vi "calculator.vi"() -> ()   [LabVIEW 2017]
panel:
  in  "QIUET":bool
  in  "*":bool
  in  "MC":bool
  in  "MR":bool
  in  "M+":bool
  in  "MS":bool
  in  "1/X":bool
  in  "+/-":bool
  in  "sqt":bool
  in  ".":bool
  out "INPUT/OUTPUT":string
  in  "b":bool
  in  "c":bool
  in  "/":bool
  in  "-":bool
  in  "+":bool
  in  "0":bool
  in  "9":bool
  in  "6":bool
  in  "8":bool
  in  "5":bool
  in  "7":bool
  in  "4":bool
  in  "3":bool
  in  "2":bool
  in  "1":bool
  in  "=":bool
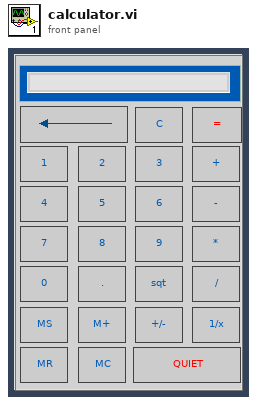
[diagram p1: front panel]
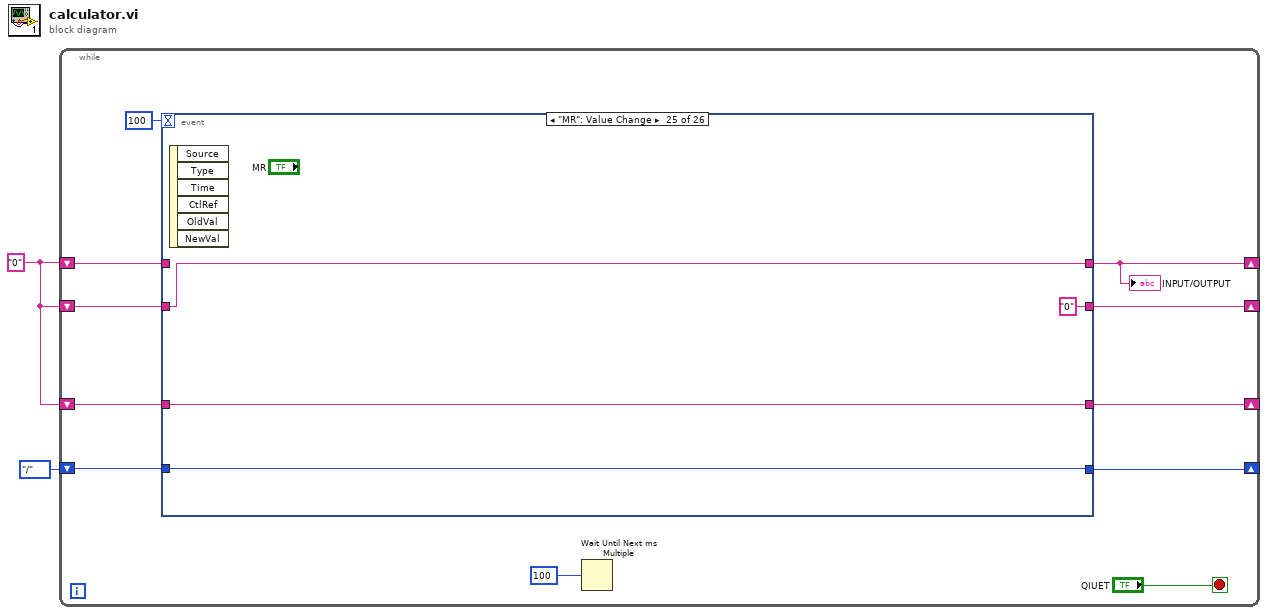
[diagram p0: block diagram]
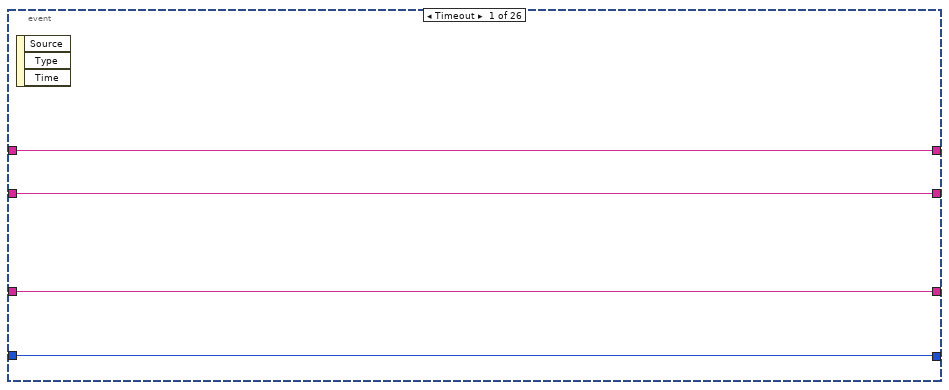
[diagram p2: hidden frame]
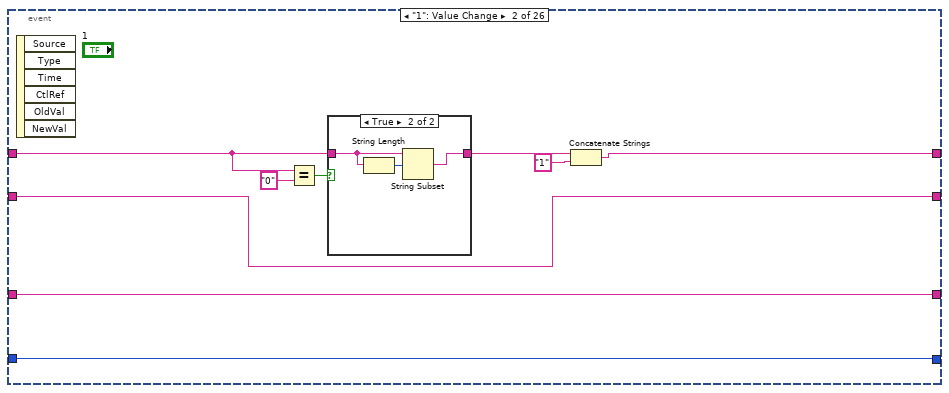
[diagram p3: hidden frame]
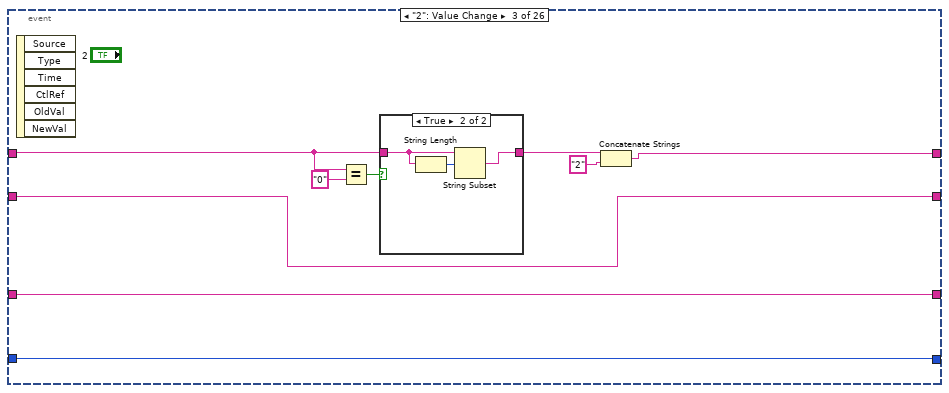
[diagram p5: hidden frame]
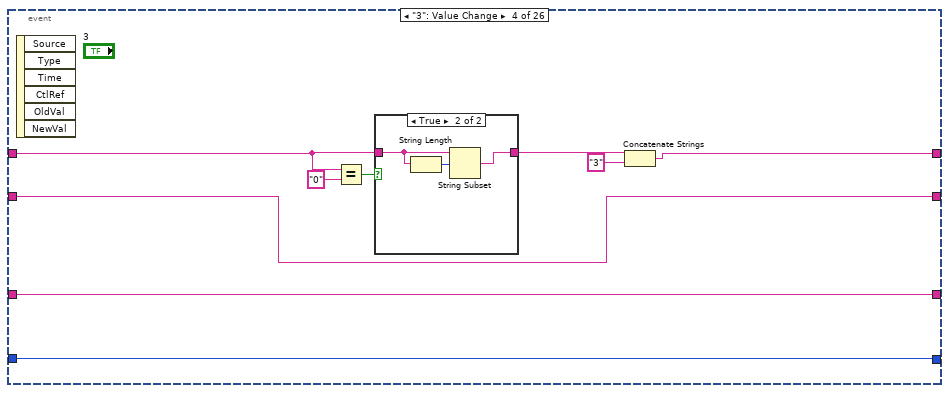
[diagram p7: hidden frame]
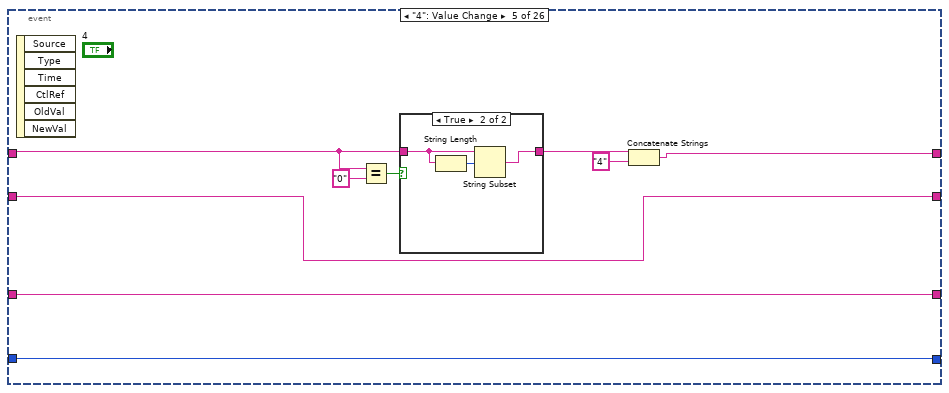
[diagram p9: hidden frame]
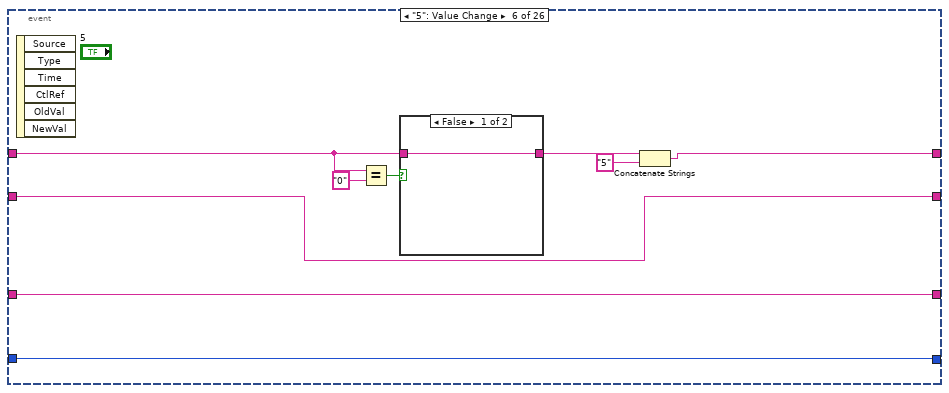
[diagram p11: hidden frame]
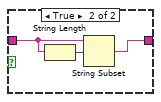
[diagram p12: hidden frame]
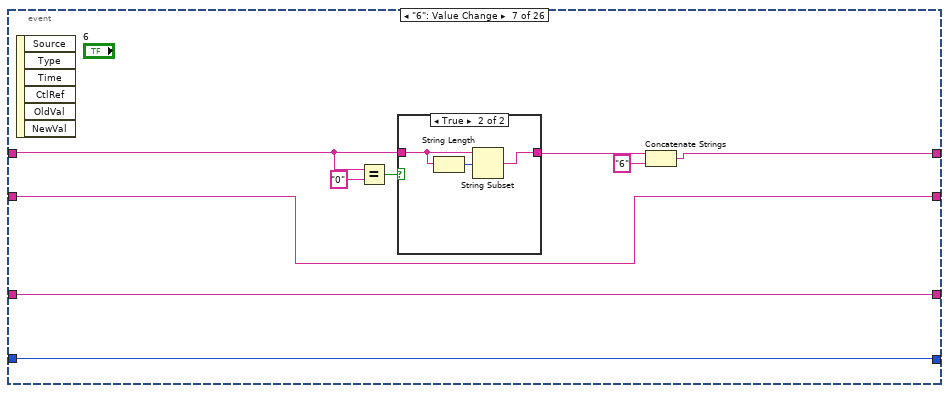
[diagram p13: hidden frame]
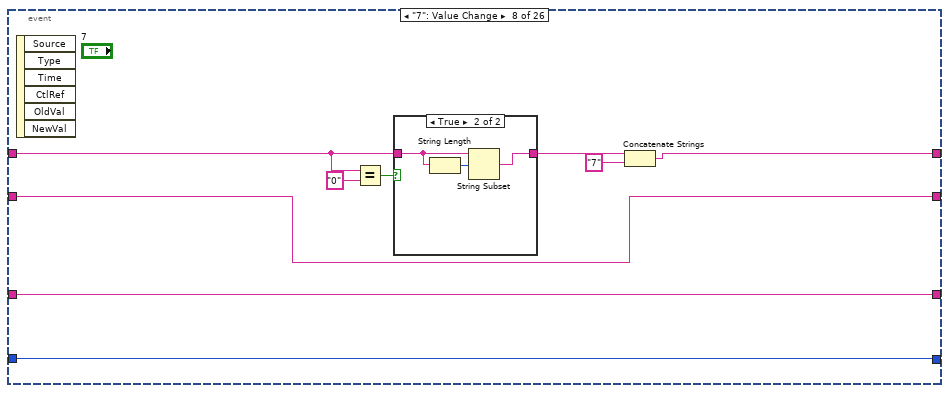
[diagram p15: hidden frame]
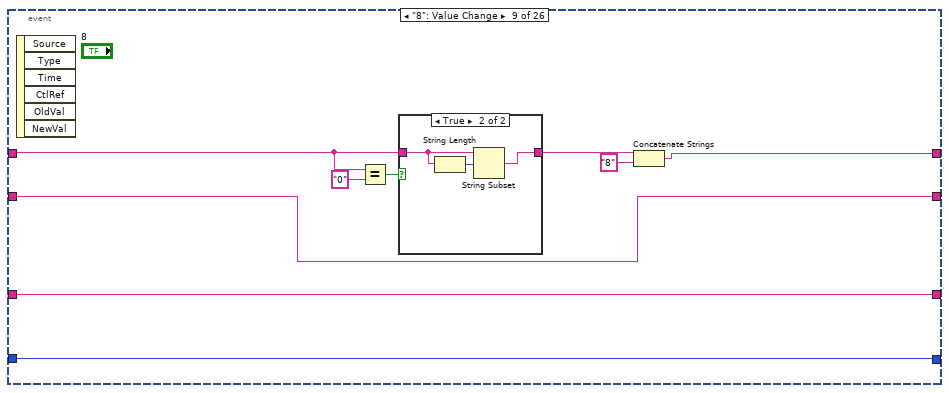
[diagram p17: hidden frame]
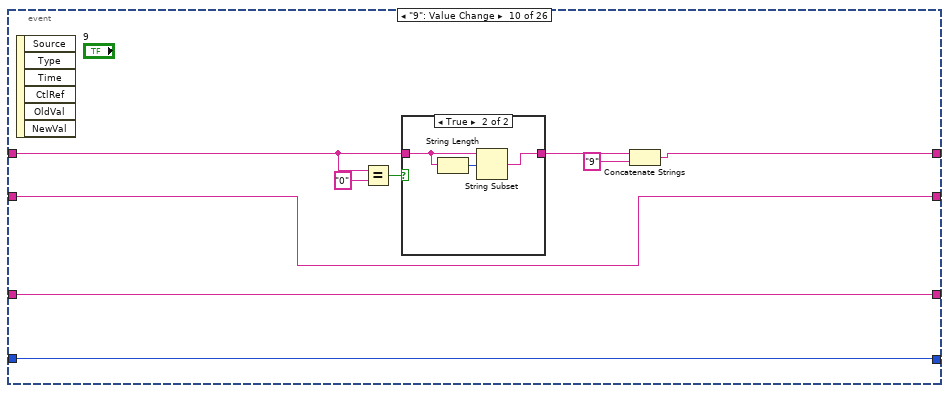
[diagram p19: hidden frame]
diagram:
  w1 = "0"
  n1 = while {
    shift-right: [w6] -> _
    shift-left: w1 -> [w13]
    shift-right: [w12] -> _
    shift-left: w1 -> [w11]
    shift-right: [w8] -> _
    shift-left: enum16{"+", "-", "*", "/"}."/" -> [w7]
    shift-right: [w5] -> _
    shift-left: w1 -> [w4]
    stop <- "QIUET" stop-if-true
    n2 = event shown="[24] \"MR\": Value Change" {
      selector: _ -> [_ _ _ _ _ _ _ _ _ _ _ _ _ _ _ _ _ _ _ _ _ _ _ _ _ _]
      dyn-events: _ -> [_ _ _ _ _ _ _ _ _ _ _ _ _ _ _ _ _ _ _ _ _ _ _ _ _ _]
      timeout: 100 -> [_ _ _ _ _ _ _ _ _ _ _ _ _ _ _ _ _ _ _ _ _ _ _ _ _ _]
      tunnel: w13 -> [w15 w19 w32 w45 w59 w71 w84 w97 w110 w123 w140 w141 w153 w157 w160 w164 w168 w177 w242 w272 w282 w317 w342 w350 _ _]
      tunnel: [w17 w25 w38 w51 w64 w77 w91 w103 w116 w129 w138 w143 w148 w157 w160 w164 w168 "0" w238 w274 w283 w314 w341 w344 w381 w384] -> w12
      tunnel: w11 -> [w17 w25 w38 w51 w64 w77 w91 w103 w116 w129 w138 w143 w148 _ _ _ _ w170 w238 w274 w283 w314 w341 w344 w381 w384]
      tunnel: w7 -> [w16 w24 w37 w50 w63 w76 w90 w102 w115 w128 w137 w144 w147 _ _ _ _ w179 w239 w273 _ _ _ w343 w380 w383]
      tunnel: [w16 w24 w37 w50 w63 w76 w90 w102 w115 w128 w137 w144 w147 enum16{"+", "-", "*", "/"}."+" enum16{"+", "-", "*", "/"}."-" enum16{"+", "-", "*", "/"}."*" enum16{"+", "-", "*", "/"}."/" w178 w239 w273 _ _ _ w343 w380 w383] -> w8
      tunnel: [w15 w23 w36 w49 w62 w75 w89 w101 w114 w127 w136 "0" w146 "0" "0" "0" "0" w173 w235 w271 w276 w310 w342 w345 w382 "0"] -> w6
      tunnel: [w14 w18 w31 w44 w57 w70 w83 w96 w109 w122 w135 w141 w145 w154 w158 w162 w166 w172 w233 w269 w275 w309 w342 _ "0" w385] -> w5
      tunnel: w4 -> [w14 w18 w31 w44 w57 w70 w83 w96 w109 w122 w135 _ w145 w154 w158 w162 w166 w172 w233 w269 w275 w309 _ w351 w382 w385]
      event Timeout {
        n3 = event-data() -> ()  [unwired: 1 in, 3 out]
      }
      event "1": Value Change {
        n4 = event-data() -> ()  [unwired: 1 in, 6 out]
        n5 = Equal?(x=w19, y="0") -> (x = y?=w22:bool)
        n6 = case shown="True" w22 {
          tunnel: w19 -> [w27 w29]
          tunnel: [w27 w28] -> w20
          frame False {
          }
          frame True {
            n7 = String Length(string=w29) -> (length=w30:i32)
            n8 = String Subset(string=w29, offset (0)=w30) -> (substring=w28:string)  [unwired: 1 in]
          }
        }
        n9 = Concatenate Strings(w20, "1") -> (w23:string)
      }
      event "2": Value Change {
        n10 = event-data() -> ()  [unwired: 1 in, 6 out]
        n11 = Equal?(x=w32, y="0") -> (x = y?=w35:bool)
        n12 = case shown="True" w35 {
          tunnel: w32 -> [w40 w42]
          tunnel: [w40 w41] -> w33
          frame False {
          }
          frame True {
            n13 = String Length(string=w42) -> (length=w43:i32)
            n14 = String Subset(string=w42, offset (0)=w43) -> (substring=w41:string)  [unwired: 1 in]
          }
        }
        n15 = Concatenate Strings(w33, "2") -> (w36:string)
      }
      event "3": Value Change {
        n16 = event-data() -> ()  [unwired: 1 in, 6 out]
        n17 = Equal?(x=w45, y="0") -> (x = y?=w48:bool)
        n18 = case shown="True" w48 {
          tunnel: w45 -> [w53 w55]
          tunnel: [w53 w54] -> w46
          frame False {
          }
          frame True {
            n19 = String Length(string=w55) -> (length=w56:i32)
            n20 = String Subset(string=w55, offset (0)=w56) -> (substring=w54:string)  [unwired: 1 in]
          }
        }
        n21 = Concatenate Strings(w46, "3") -> (w49:string)
      }
      event "4": Value Change {
        n22 = event-data() -> ()  [unwired: 1 in, 6 out]
        n23 = Equal?(x=w59, y="0") -> (x = y?=w61:bool)
        n24 = case shown="True" w61 {
          tunnel: w59 -> [w66 w68]
          tunnel: [w66 w67] -> w58
          frame False {
          }
          frame True {
            n25 = String Length(string=w68) -> (length=w69:i32)
            n26 = String Subset(string=w68, offset (0)=w69) -> (substring=w67:string)  [unwired: 1 in]
          }
        }
        n27 = Concatenate Strings(w58, "4") -> (w62:string)
      }
      event "5": Value Change {
        n28 = event-data() -> ()  [unwired: 1 in, 6 out]
        n29 = Equal?(x=w71, y="0") -> (x = y?=w74:bool)
        n30 = case shown="False" w74 {
          tunnel: w71 -> [w79 w81]
          tunnel: [w79 w80] -> w72
          frame False {
          }
          frame True {
            n31 = String Length(string=w81) -> (length=w82:i32)
            n32 = String Subset(string=w81, offset (0)=w82) -> (substring=w80:string)  [unwired: 1 in]
          }
        }
        n33 = Concatenate Strings(w72, "5") -> (w75:string)
      }
      event "6": Value Change {
        n34 = event-data() -> ()  [unwired: 1 in, 6 out]
        n35 = Equal?(x=w84, y="0") -> (x = y?=w87:bool)
        n36 = case shown="True" w87 {
          tunnel: w84 -> [w92 w94]
          tunnel: [w92 w93] -> w85
          frame False {
          }
          frame True {
            n37 = String Length(string=w94) -> (length=w95:i32)
            n38 = String Subset(string=w94, offset (0)=w95) -> (substring=w93:string)  [unwired: 1 in]
          }
        }
        n39 = Concatenate Strings(w85, "6") -> (w89:string)
      }
      event "7": Value Change {
        n40 = event-data() -> ()  [unwired: 1 in, 6 out]
        n41 = Equal?(x=w97, y="0") -> (x = y?=w100:bool)
        n42 = case shown="True" w100 {
          tunnel: w97 -> [w105 w107]
          tunnel: [w105 w106] -> w98
          frame False {
          }
          frame True {
            n43 = String Length(string=w107) -> (length=w108:i32)
            n44 = String Subset(string=w107, offset (0)=w108) -> (substring=w106:string)  [unwired: 1 in]
          }
        }
        n45 = Concatenate Strings(w98, "7") -> (w101:string)
      }
      event "8": Value Change {
        n46 = event-data() -> ()  [unwired: 1 in, 6 out]
        n47 = Equal?(x=w110, y="0") -> (x = y?=w113:bool)
        n48 = case shown="True" w113 {
          tunnel: w110 -> [w118 w120]
          tunnel: [w118 w119] -> w111
          frame False {
          }
          frame True {
            n49 = String Length(string=w120) -> (length=w121:i32)
            n50 = String Subset(string=w120, offset (0)=w121) -> (substring=w119:string)  [unwired: 1 in]
          }
        }
        n51 = Concatenate Strings(w111, "8") -> (w114:string)
      }
      event "9": Value Change {
        n52 = event-data() -> ()  [unwired: 1 in, 6 out]
        n53 = Equal?(x=w123, y="0") -> (x = y?=w126:bool)
        n54 = case shown="True" w126 {
          tunnel: w123 -> [w131 w133]
          tunnel: [w131 w132] -> w124
          frame False {
          }
          frame True {
            n55 = String Length(string=w133) -> (length=w134:i32)
            n56 = String Subset(string=w133, offset (0)=w134) -> (substring=w132:string)  [unwired: 1 in]
          }
        }
        n57 = Concatenate Strings(w124, "9") -> (w127:string)
      }
      event "0": Value Change {
        n58 = event-data() -> ()  [unwired: 1 in, 6 out]
        n59 = Concatenate Strings(w140, "0") -> (w136:string)
      }
      event "c": Value Change {
        n60 = event-data() -> ()  [unwired: 1 in, 6 out]
      }
      event "b": Value Change {
        n61 = event-data() -> ()  [unwired: 1 in, 6 out]
        n62 = Reverse String(1:w153) -> (0:w149:string)
        n63 = String Length(string=w149) -> (length=w150:i32)
        n64 = String Subset(string=w149, offset (0)=1, length (rest)=w150) -> (substring=w151:string)
        n65 = Reverse String(1:w151) -> (0:w146:string)
      }
      event "+": Value Change {
        n66 = event-data() -> ()  [unwired: 1 in, 6 out]
      }
      event "-": Value Change {
        n67 = event-data() -> ()  [unwired: 1 in, 6 out]
      }
      event "*": Value Change {
        n68 = event-data() -> ()  [unwired: 1 in, 6 out]
      }
      event "/": Value Change {
        n69 = event-data() -> ()  [unwired: 1 in, 6 out]
      }
      event "=": Value Change {
        n70 = event-data() -> ()  [unwired: 1 in, 6 out]
        n71 = case shown="\"-\"" w179 {
          selector: w179 -> [w211 w218 w225 w232]
          tunnel: [w211 w218 w225 w232] -> w178
          tunnel: w170 -> [w207 w213 w220 w227]
          tunnel: w177 -> [w206 w214 w221 w228]
          tunnel: [w205 w212 w219 w226] -> w174
          frame "+" {
            n72 = Fract/Exp String To Number(string=w206) -> (number=w209:dbl)  [unwired: 3 in, 1 out]
            n73 = Fract/Exp String To Number(string=w207) -> (number=w210:dbl)  [unwired: 3 in, 1 out]
            n74 = Add(x=w210, y=w209) -> (x+y=w208:dbl)
            n75 = Number To Fractional String(number=w208) -> (F-format string=w205:string)  [unwired: 3 in]
          }
          frame "-" {
            n76 = Fract/Exp String To Number(string=w214) -> (number=w216:dbl)  [unwired: 3 in, 1 out]
            n77 = Fract/Exp String To Number(string=w213) -> (number=w217:dbl)  [unwired: 3 in, 1 out]
            n78 = Subtract(x=w217, y=w216) -> (x-y=w215:dbl)
            n79 = Number To Fractional String(number=w215) -> (F-format string=w212:string)  [unwired: 3 in]
          }
          frame "*" {
            n80 = Fract/Exp String To Number(string=w221) -> (number=w223:dbl)  [unwired: 3 in, 1 out]
            n81 = Fract/Exp String To Number(string=w220) -> (number=w224:dbl)  [unwired: 3 in, 1 out]
            n82 = Multiply(x=w224, y=w223) -> (x*y=w222:dbl)
            n83 = Number To Fractional String(number=w222) -> (F-format string=w219:string)  [unwired: 3 in]
          }
          frame "/" {
            n84 = Fract/Exp String To Number(string=w228) -> (number=w230:dbl)  [unwired: 3 in, 1 out]
            n85 = Fract/Exp String To Number(string=w227) -> (number=w231:dbl)  [unwired: 3 in, 1 out]
            n86 = Divide(x=w231, y=w230) -> (x/y=w229:dbl)
            n87 = Number To Fractional String(number=w229) -> (F-format string=w226:string)  [unwired: 3 in]
          }
        }
        n88 = String Length(string=w174) -> (length=w176:i32)
        n89 = for {
          N: w176 -> [_]
          tunnel: w174 -> [w189]
          shift-right: [w188] -> _
          shift-left: "" -> [w192]
          tunnel: [w181] -> w173
          i -> [w194]
          stop <- w183 stop-if-true
          n90 = Reverse String(1:w189) -> (0:w190:string)
          n91 = String Subset(string=w190, offset (0)=w194, length (rest)=1 ("length (rest)")) -> (substring=w186:string)
          n92 = Greater?(x=w186, y="0") -> (0:w184:bool)
          n93 = Equal?(x=w186, y=".") -> (x = y?=w180:bool)
          n94 = Or(x=w180, y=w184) -> (x .or. y?=w183:bool)
          n95 = case shown="True" w183 {
            tunnel: w192 -> [w203 w204]
            tunnel: w186 -> [w202 _]
            tunnel: [w201 w204] -> w188
            frame False {
              n96 = Concatenate Strings(w203, w202) -> (w201:string)
            }
            frame True {
            }
          }
          n97 = Reverse String(1:w188) -> (0:w187:string)
          n98 = Match Pattern(string=w189, regular expression=w187) -> (before substring=w182:string)  [unwired: 1 in, 3 out]
          n99 = case shown="True" w180 {
            tunnel: w182 -> [w195 w200]
            tunnel: [w195 w196] -> w181
            frame False {
            }
            frame True {
              n100 = Reverse String(1:w200) -> (0:w198:string)
              n101 = Match Pattern(string=w198, regular expression=".") -> (after substring=w197:string)  [unwired: 1 in, 3 out]
              n102 = Reverse String(1:w197) -> (0:w196:string)
            }
          }
        }
      }
      event "sqt": Value Change {
        n103 = event-data() -> ()  [unwired: 1 in, 6 out]
        n104 = Fract/Exp String To Number(string=w242) -> (number=w241:dbl)  [unwired: 3 in, 1 out]
        n105 = Square Root(x=w241) -> (sqrt(x)=w240:dbl)
        n106 = Number To Fractional String(number=w240) -> (F-format string=w234:string)  [unwired: 3 in]
        n107 = String Length(string=w234) -> (length=w237:i32)
        n108 = for {
          N: w237 -> [_]
          tunnel: w234 -> [w253]
          shift-right: [w252] -> _
          shift-left: "" -> [w256]
          tunnel: [w245] -> w235
          tunnel: w234 -> [w243]
          i -> [w258]
          stop <- w247 stop-if-true
          n109 = Reverse String(1:w253) -> (0:w254:string)
          n110 = String Subset(string=w254, offset (0)=w258, length (rest)=1 ("length (rest)")) -> (substring=w250:string)
          n111 = Greater?(x=w250, y="0") -> (0:w248:bool)
          n112 = Equal?(x=w250, y=".") -> (x = y?=w244:bool)
          n113 = Or(x=w244, y=w248) -> (x .or. y?=w247:bool)
          n114 = case shown="True" w247 {
            tunnel: w256 -> [w267 w268]
            tunnel: w250 -> [w266 _]
            tunnel: [w265 w268] -> w252
            frame False {
              n115 = Concatenate Strings(w267, w266) -> (w265:string)
            }
            frame True {
            }
          }
          n116 = Reverse String(1:w252) -> (0:w251:string)
          n117 = Match Pattern(string=w253, regular expression=w251) -> (before substring=w246:string)  [unwired: 1 in, 3 out]
          n118 = case shown="True" w244 {
            tunnel: w246 -> [_ w264]
            tunnel: [w259 w260] -> w245
            tunnel: w243 -> [w259 _]
            frame False {
            }
            frame True {
              n119 = Reverse String(1:w264) -> (0:w262:string)
              n120 = Match Pattern(string=w262, regular expression=".") -> (after substring=w261:string)  [unwired: 1 in, 3 out]
              n121 = Reverse String(1:w261) -> (0:w260:string)
            }
          }
        }
      }
      event ".": Value Change {
        n122 = event-data() -> ()  [unwired: 1 in, 6 out]
        n123 = Concatenate Strings(w272, "." ("string")) -> (w271:string)
      }
      event "+/-": Value Change {
        n124 = event-data() -> ()  [unwired: 1 in, 6 out]
        n125 = Fract/Exp String To Number(string=w282) -> (number=w281:dbl)  [unwired: 3 in, 1 out]
        n126 = Negate(x=w281) -> (-x=w280:dbl)
        n127 = Number To Fractional String(number=w280) -> (F-format string=w277:string)  [unwired: 3 in]
        n128 = String Length(string=w277) -> (length=w279:i32)
        n129 = for {
          N: w279 -> [_]
          tunnel: w277 -> [w293]
          shift-right: [w292] -> _
          shift-left: "" -> [w296]
          tunnel: [w285] -> w276
          i -> [w298]
          stop <- w287 stop-if-true
          n130 = Reverse String(1:w293) -> (0:w294:string)
          n131 = String Subset(string=w294, offset (0)=w298, length (rest)=1 ("length (rest)")) -> (substring=w290:string)
          n132 = Greater?(x=w290, y="0") -> (0:w288:bool)
          n133 = Equal?(x=w290, y=".") -> (x = y?=w284:bool)
          n134 = Or(x=w284, y=w288) -> (x .or. y?=w287:bool)
          n135 = case shown="True" w287 {
            tunnel: w296 -> [w307 w308]
            tunnel: w290 -> [w306 _]
            tunnel: [w305 w308] -> w292
            frame False {
              n136 = Concatenate Strings(w307, w306) -> (w305:string)
            }
            frame True {
            }
          }
          n137 = Reverse String(1:w292) -> (0:w291:string)
          n138 = Match Pattern(string=w293, regular expression=w291) -> (before substring=w286:string)  [unwired: 1 in, 3 out]
          n139 = case shown="True" w284 {
            tunnel: w286 -> [w299 w304]
            tunnel: [w299 w300] -> w285
            frame False {
            }
            frame True {
              n140 = Reverse String(1:w304) -> (0:w302:string)
              n141 = Match Pattern(string=w302, regular expression=".") -> (after substring=w301:string)  [unwired: 1 in, 3 out]
              n142 = Reverse String(1:w301) -> (0:w300:string)
            }
          }
        }
      }
      event "1/X": Value Change {
        n143 = event-data() -> ()  [unwired: 1 in, 6 out]
        n144 = Fract/Exp String To Number(string=w317) -> (number=w316:dbl)  [unwired: 3 in, 1 out]
        n145 = Reciprocal(x=w316) -> (1/x=w315:dbl)
        n146 = Number To Fractional String(number=w315) -> (F-format string=w311:string)  [unwired: 3 in]
        n147 = String Length(string=w311) -> (length=w313:i32)
        n148 = for {
          N: w313 -> [_]
          tunnel: w311 -> [w320]
          shift-right: [w319] -> _
          shift-left: "" -> [w327]
          tunnel: [w318] -> w310
          i -> [w329]
          stop <- w323 stop-if-true
          n149 = Reverse String(1:w320) -> (0:w325:string)
          n150 = String Subset(string=w325, offset (0)=w329, length (rest)=1 ("length (rest)")) -> (substring=w324:string)
          n151 = Greater?(x=w324, y="0") -> (0:w323:bool)
          n152 = case shown="True" w323 {
            tunnel: w327 -> [w339 w340]
            tunnel: w324 -> [w338 _]
            tunnel: [w337 w340] -> w319
            frame False {
              n153 = Concatenate Strings(w339, w338) -> (w337:string)
            }
            frame True {
            }
          }
          n154 = Equal?(x=w319, y="") -> (x = y?=w322:bool)
          n155 = case shown="True" w322 {
            tunnel: w320 -> [w333 w336]
            tunnel: w319 -> [w332 _]
            tunnel: [w330 w334] -> w318
            frame False {
              n156 = Reverse String(1:w332) -> (0:w331:string)
              n157 = Match Pattern(string=w333, regular expression=w331) -> (before substring=w330:string)  [unwired: 1 in, 3 out]
            }
            frame True {
              n158 = call <vilib>:"Space Constant.vi"() -> ("String"=w335:string)
              n159 = Match Pattern(string=w336, regular expression=w335) -> (before substring=w334:string)  [unwired: 1 in, 3 out]
            }
          }
        }
      }
      event "MS": Value Change {
        n160 = event-data() -> ()  [unwired: 1 in, 6 out]
      }
      event "M+": Value Change {
        n161 = event-data() -> ()  [unwired: 1 in, 6 out]
        n162 = Fract/Exp String To Number(string=w350) -> (number=w348:dbl)  [unwired: 3 in, 1 out]
        n163 = Fract/Exp String To Number(string=w351) -> (number=w349:dbl)  [unwired: 3 in, 1 out]
        n164 = Add(x=w349, y=w348) -> (x+y=w347:dbl)
        n165 = Number To Fractional String(number=w347) -> (F-format string=w346:string)  [unwired: 3 in]
        n166 = String Length(string=w346) -> (length=w353:i32)
        n167 = for {
          N: w353 -> [_]
          tunnel: w346 -> [w363]
          shift-right: [w362] -> _
          shift-left: "" -> [w366]
          tunnel: [w355] -> w345
          i -> [w368]
          stop <- w357 stop-if-true
          n168 = Reverse String(1:w363) -> (0:w364:string)
          n169 = String Subset(string=w364, offset (0)=w368, length (rest)=1 ("length (rest)")) -> (substring=w360:string)
          n170 = Greater?(x=w360, y="0") -> (0:w358:bool)
          n171 = Equal?(x=w360, y=".") -> (x = y?=w354:bool)
          n172 = Or(x=w354, y=w358) -> (x .or. y?=w357:bool)
          n173 = case shown="False" w357 {
            tunnel: w366 -> [w377 w378]
            tunnel: w360 -> [w376 _]
            tunnel: [w375 w378] -> w362
            frame False {
              n174 = Concatenate Strings(w377, w376) -> (w375:string)
            }
            frame True {
            }
          }
          n175 = Reverse String(1:w362) -> (0:w361:string)
          n176 = Match Pattern(string=w363, regular expression=w361) -> (before substring=w356:string)  [unwired: 1 in, 3 out]
          n177 = case shown="False" w354 {
            tunnel: w356 -> [w369 w374]
            tunnel: [w369 w370] -> w355
            frame False {
            }
            frame True {
              n178 = Reverse String(1:w374) -> (0:w372:string)
              n179 = Match Pattern(string=w372, regular expression=".") -> (after substring=w371:string)  [unwired: 1 in, 3 out]
              n180 = Reverse String(1:w371) -> (0:w370:string)
            }
          }
        }
      }
      event "MR": Value Change {
        n181 = event-data() -> ()  [unwired: 1 in, 6 out]
      }
      event "MC": Value Change {
        n182 = event-data() -> ()  [unwired: 1 in, 6 out]
      }
    }
    "INPUT/OUTPUT" <- w6
    n183 = Wait Until Next ms Multiple(millisecond multiple=u32 100) -> ()  [unwired: 1 out]
  }
